vi "LED intensity controlling.vi"() -> ()   [LabVIEW 2022 SP3]
panel:
  in  "VISA Refnum in 3":refnum<visa-resource-name>
  in  "VISA Refnum in 2":refnum<visa-resource-name>
  in  "VISA Refnum in":refnum<visa-resource-name>
  in  "Numeric":dbl
  in  "stop":bool
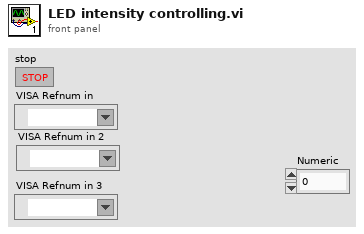
[diagram p1: front panel]
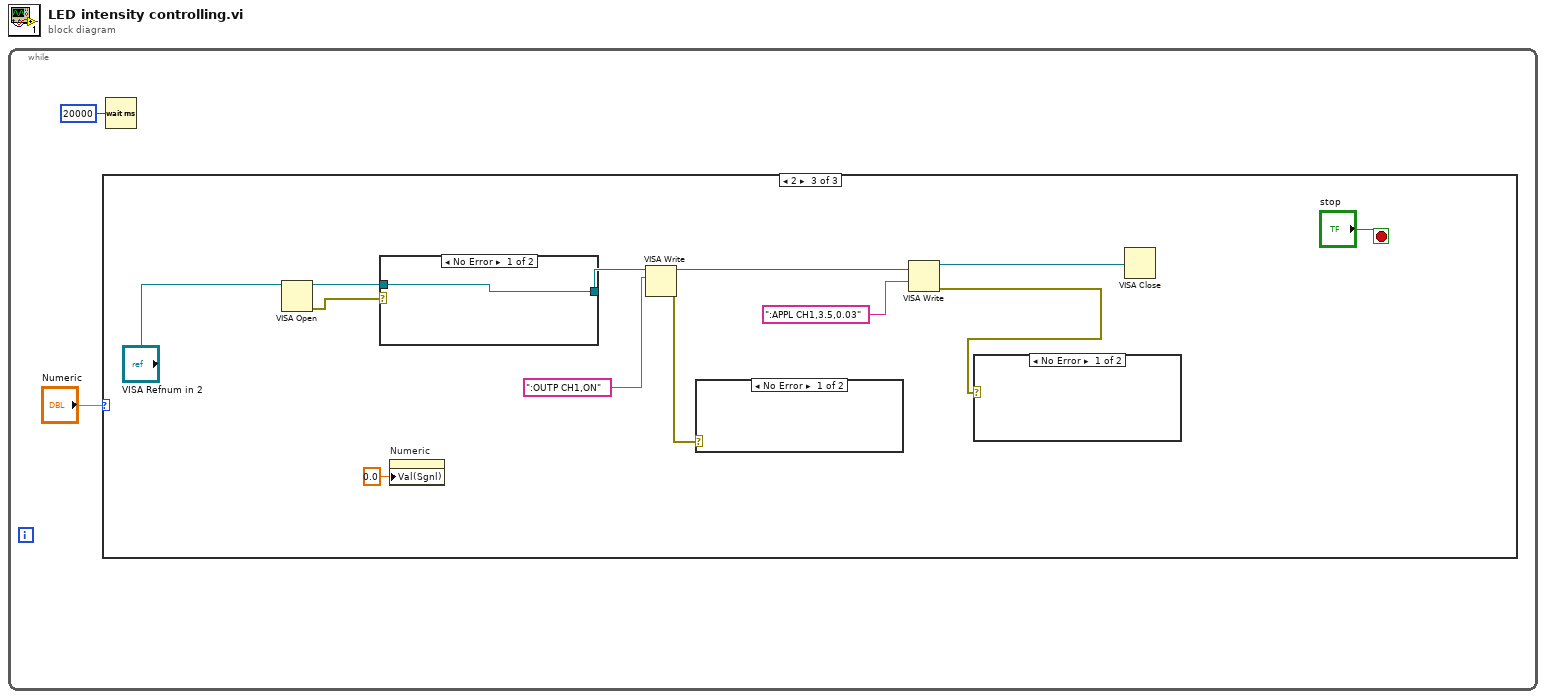
[diagram p0: block diagram]
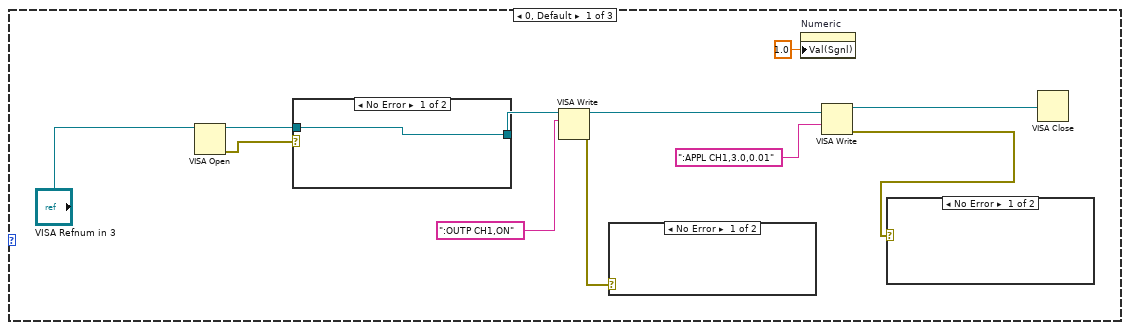
[diagram p2: hidden frame]
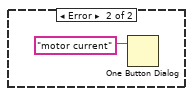
[diagram p3: hidden frame]
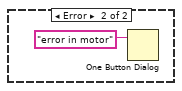
[diagram p4: hidden frame]
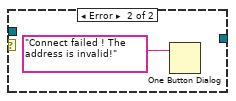
[diagram p5: hidden frame]
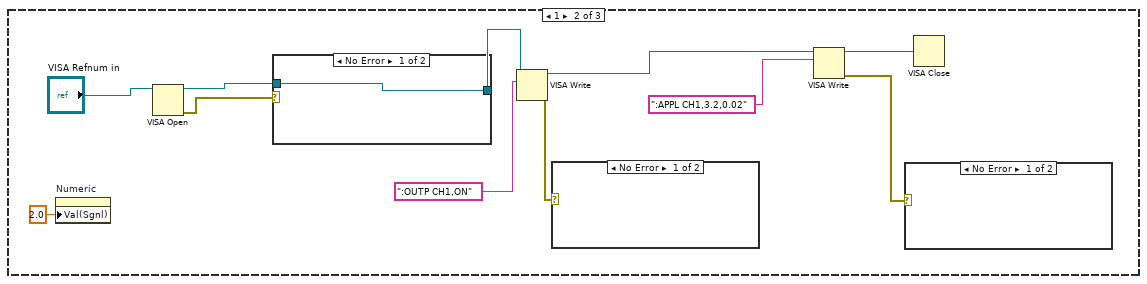
[diagram p6: hidden frame]
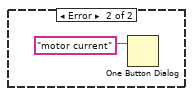
[diagram p7: hidden frame]
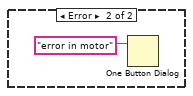
[diagram p8: hidden frame]
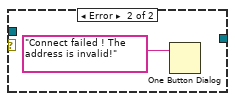
[diagram p9: hidden frame]
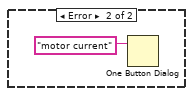
[diagram p10: hidden frame]
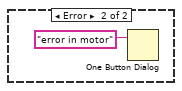
[diagram p11: hidden frame]
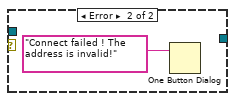
[diagram p12: hidden frame]
diagram:
  n1 = while {
    stop <- "stop" stop-if-true
    n2 = case shown="2" "Numeric" {
      frame 0, Default {
        n3 = VISA Open(VISA resource name="VISA Refnum in 3") -> (VISA resource name=w11:refnum<visa-resource-name>, error out=w10:errorcluster)  [unwired: 4 in]
        n4 = case shown="No Error" w10 {
          tunnel: w11 -> [w17 _]
          tunnel: [w17 _] -> w8
          frame No Error {
          }
          frame Error {
            n5 = One Button Dialog(message="Connect failed ! The address is invalid!") -> ()  [unwired: 1 in, 1 out]
          }
        }
        n6 = VISA Write(VISA resource name=w8, write buffer=":OUTP CH1,ON") -> (VISA resource name out=w5:refnum<visa-resource-name>, error out=w6:errorcluster)  [unwired: 1 in, 1 out]
        n7 = case shown="No Error" w6 {
          frame No Error {
          }
          frame Error {
            n8 = One Button Dialog(message="error in motor") -> ()  [unwired: 1 in, 1 out]
          }
        }
        n9 = property on="Numeric" class="DigNum (strict)"("Val(Sgnl)"=1.0 ("Value (Signaling)")) -> ()  [unwired: 2 in, 2 out]
        n10 = VISA Write(VISA resource name=w5, write buffer=":APPL CH1,3.0,0.01") -> (VISA resource name out=w12:refnum<visa-resource-name>, error out=w4:errorcluster)  [unwired: 1 in, 1 out]
        n11 = case shown="No Error" w4 {
          frame No Error {
          }
          frame Error {
            n12 = One Button Dialog(message="motor current") -> ()  [unwired: 1 in, 1 out]
          }
        }
        n13 = VISA Close(VISA resource name=w12) -> ()  [unwired: 1 in, 1 out]
      }
      frame 1 {
        n14 = property on="Numeric" class="DigNum (strict)"("Val(Sgnl)"=2.0 ("Value (Signaling)")) -> ()  [unwired: 2 in, 2 out]
        n15 = VISA Open(VISA resource name="VISA Refnum in") -> (VISA resource name=w27:refnum<visa-resource-name>, error out=w26:errorcluster)  [unwired: 4 in]
        n16 = case shown="No Error" w26 {
          tunnel: w27 -> [w32 _]
          tunnel: [w32 _] -> w25
          frame No Error {
          }
          frame Error {
            n17 = One Button Dialog(message="Connect failed ! The address is invalid!") -> ()  [unwired: 1 in, 1 out]
          }
        }
        n18 = VISA Write(VISA resource name=w25, write buffer=":OUTP CH1,ON") -> (VISA resource name out=w22:refnum<visa-resource-name>, error out=w23:errorcluster)  [unwired: 1 in, 1 out]
        n19 = case shown="No Error" w23 {
          frame No Error {
          }
          frame Error {
            n20 = One Button Dialog(message="error in motor") -> ()  [unwired: 1 in, 1 out]
          }
        }
        n21 = VISA Write(VISA resource name=w22, write buffer=":APPL CH1,3.2,0.02") -> (VISA resource name out=w28:refnum<visa-resource-name>, error out=w21:errorcluster)  [unwired: 1 in, 1 out]
        n22 = case shown="No Error" w21 {
          frame No Error {
          }
          frame Error {
            n23 = One Button Dialog(message="motor current") -> ()  [unwired: 1 in, 1 out]
          }
        }
        n24 = VISA Close(VISA resource name=w28) -> ()  [unwired: 1 in, 1 out]
      }
      frame 2 {
        n25 = VISA Open(VISA resource name="VISA Refnum in 2") -> (VISA resource name=w42:refnum<visa-resource-name>, error out=w41:errorcluster)  [unwired: 4 in]
        n26 = case shown="No Error" w41 {
          tunnel: w42 -> [w47 _]
          tunnel: [w47 _] -> w39
          frame No Error {
          }
          frame Error {
            n27 = One Button Dialog(message="Connect failed ! The address is invalid!") -> ()  [unwired: 1 in, 1 out]
          }
        }
        n28 = property on="Numeric" class="DigNum (strict)"("Val(Sgnl)"=0.0 ("Value (Signaling)")) -> ()  [unwired: 2 in, 2 out]
        n29 = VISA Write(VISA resource name=w39, write buffer=":OUTP CH1,ON") -> (VISA resource name out=w36:refnum<visa-resource-name>, error out=w37:errorcluster)  [unwired: 1 in, 1 out]
        n30 = case shown="No Error" w37 {
          frame No Error {
          }
          frame Error {
            n31 = One Button Dialog(message="error in motor") -> ()  [unwired: 1 in, 1 out]
          }
        }
        n32 = VISA Write(VISA resource name=w36, write buffer=":APPL CH1,3.5,0.03") -> (VISA resource name out=w43:refnum<visa-resource-name>, error out=w35:errorcluster)  [unwired: 1 in, 1 out]
        n33 = case shown="No Error" w35 {
          frame No Error {
          }
          frame Error {
            n34 = One Button Dialog(message="motor current") -> ()  [unwired: 1 in, 1 out]
          }
        }
        n35 = VISA Close(VISA resource name=w43) -> ()  [unwired: 1 in, 1 out]
      }
    }
    n36 = Wait (ms)(milliseconds to wait=u32 20000) -> ()  [unwired: 1 out]
  }
